vi "Teleop.vi"(10 "Match Info":T2={"Autonomous Elapsed Seconds"=0.0, "TeleOp Elapsed Seconds"=0.0, "Disabled Elapsed Seconds"=0.0, "Visited Autonomous"=FALSE, "Visited TeleOp"=FALSE, "Visited Disabled"=FALSE, "Autonomous Settings"={"Autonomous Style"=enum."Independent", "VI Refnum"=refnum}}, 11 "Call Context":T3) -> ()   [LabVIEW 2019]
doc: "This VI is called for each TeleOp packet received from the DS where the robot is not disabled. It is often used to read from the joysticks and update I/O or to update setpoints for timed control loops. It should complete and return within 20 milliseconds or it may miss DS packets."
uses:
  <vilib>/Rock Robotics/WPI/DriverStation/WPI_DriverStationDerivedRobotMode.ctl
  <vilib>/Rock Robotics/WPI/DriverStation/WPI_DriverStationMatch Info.ctl
  <vilib>/Rock Robotics/WPI/Solenoid/WPI_SolenoidValue.ctl
  <vilib>/Rock Robotics/WPI/Relay/WPI_RelayValue.ctl
  <vilib>/Rock Robotics/WPI/Utilities/WPI_GetSetVariantRefNum.vi
  <vilib>/Rock Robotics/Network Tables/NT Read Boolean.vi
  <vilib>/Rock Robotics/Network Tables/NT Write Boolean.vi
  <vilib>/Rock Robotics/WPI/RobotDrive/WPI_RobotDriveMecanumDrive_Cartesian.vi
  <vilib>/Rock Robotics/WPI/Solenoid/WPI_SolenoidSetEnum.vi
panel:
  out "Right JS\nButton 4\nConveyor\nReverse":bool
  out "Left JS\nButton 3\nCW Turner R override":bool
  out "Left JS\nButton 5\nCW Turner F override":bool
  out "FMS = Green":bool
  out "FMS = Yellow":bool
  out "FMS=Red":bool
  out "FMS=Blue":bool
  out "CW Turner Distance (in)":dbl
  out "Number of Revolutions":dbl
  out "Current angle (deg)":dbl
  out "Encoder Direction":dbl
  out "Encoder Rate (deg/sec)":dbl
  out "Left JS\nButton 8\nReset Encoder":bool
  out "Right JS\nButton 6\nConveyor\nForward":bool
  out "Right JS\nButton 1\nShooter":bool
  out "Button 4\nHD Off":bool
  out "Left JS Button 7\nCW Turner":bool
  out "Left JS\nButton 1\nWinch":bool
  out "Pincher Solenoid Value":T1
  out "Pincher Button Pressed":dbl
  out "Hook Deployer Solenoid Value":T1=enum."Forward"
  out "Hook Deployer \nButton Pressed":dbl
  out "Z value":dbl
  out "Y value":dbl
  out "X value":dbl
  out "Button 11\nPincher Release":bool
  out "Button 10\nPincher Off":bool
  out "Button 7\nPincher Grab":bool
  out "Button 5\nHD Up":bool
  out "Button 3\nHD Down":bool
  # "Drive Control"
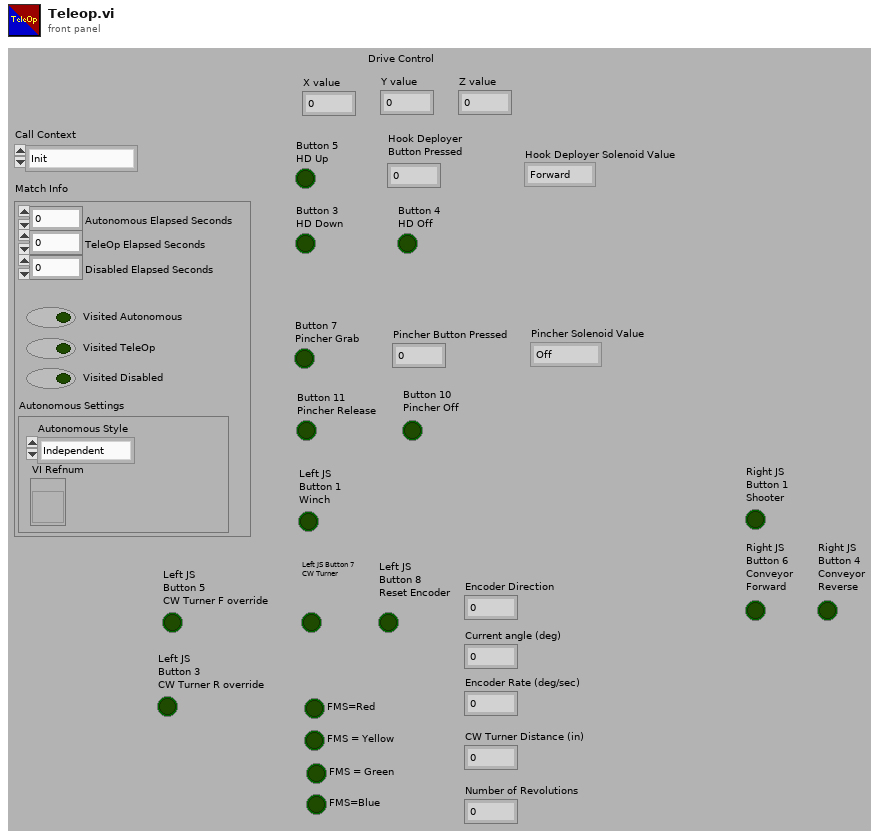
[diagram p1: front panel]
types:
  T1 = typedef "WPI_SolenoidValue.ctl" = enum16{"Off", "On", "Forward", "Reverse"}
  T2 = typedef "WPI_DriverStationMatch Info.ctl" = cluster{"Autonomous Elapsed Seconds":dbl, "TeleOp Elapsed Seconds":dbl, "Disabled Elapsed Seconds":dbl, "Visited Autonomous":bool, "Visited TeleOp":bool, "Visited Disabled":bool, "Autonomous Settings":cluster{"Autonomous Style":enum16{"Iterative", "Independent"}, "VI Refnum":refnum<vi>}}
  T3 = typedef "WPI_DriverStationDerivedRobotMode.ctl" = enum16{"Init", "Execute", "Stop"}
  T4 = typedef "WPI_EncoderDevRef.ctl" = cluster{"DevStatus":errorcluster, "EncoderIndex":T5, "CounterIndex":T6, "DistancePerCount":dbl, "Decoding Type":T7}
  T5 = typedef "FPGA_EncoderIdx.ctl" = enum8{"Enc 0", "Enc 1", "Enc 2", "Enc 3", "Enc 4", "Enc 5", "Enc 6", "Enc 7", "Invalid"}
  T6 = typedef "FPGA_CounterCtrSystemIndex.ctl" = enum8{"Ctr 0", "Ctr 1", "Ctr 2", "Ctr 3", "Ctr 4", "Ctr 5", "Ctr 6", "Ctr 7", "Invalid"}
  T7 = typedef "WPI_EncoderType.ctl" = enum16{"1x", "2x", "4x"}
  T8 = typedef "WPI_JoystickDevRef.ctl" = cluster{"Device":T9}
  T9 = typedef "WPI_JoystickDeviceEnum.ctl" = enum16{"USB 0", "USB 1", "USB 2", "USB 3", "USB 4", "USB 5"}
  T10 = typedef "WPI_RelayDevRef.ctl" = cluster{"DevStatus":errorcluster, "Relay Channel":T11, "Relay Direction":T12}
  T11 = typedef "FPGA_DIORelayChannel.ctl" = enum8{"Relay 0", "Relay 1", "Relay 2", "Relay 3", "Invalid"}
  T12 = typedef "WPI_RelayDirection.ctl" = enum16{"Both directions", "Forward only", "Reverse only"}
  T13 = typedef "WPI_RelayValue.ctl" = enum16{"Off", "On", "Forward", "Reverse"}
  T14 = typedef "WPI_MotorControlDeviceRef.ctl" = cluster{"DeviceStatus":errorcluster, "Type":T15, "PWM":cluster{"PWM Channel":T16, "DeadBand":T17}, "CAN":cluster{"Device Number":u8, "SetOutput VI Ref":variant, "GetOutput VI Ref":variant, "Enable VI Ref":variant, "Disable VI Ref":variant, "Data":variant}, "Invert":bool, "DIO PWM":cluster{"PWM \"Enable\" Channel":T16, "DIOChannel":T18, "PWM Rate":dbl}}
  T15 = typedef "WPI_MotorControlType.ctl" = enum16{"PWM", "CAN", "DIO PWM"}
  T16 = typedef "FPGA_DIOPWMChannel.ctl" = enum8{"PWM 0", "PWM 1", "PWM 2", "PWM 3", "PWM 4", "PWM 5", "PWM 6", "PWM 7", "PWM 8", "PWM 9", "PWM MXP 0", "PWM MXP 1", "PWM MXP 2", "PWM MXP 3", "PWM MXP 4", "PWM MXP 5", "PWM MXP 6", "PWM MXP 7", "PWM MXP 8", "PWM MXP 9", "Invalid"}
  T17 = typedef "WPI_PWMDeadband.ctl" = cluster{"Name":string, "maxPositivePwm":i32, "minPositivePwm":i32, "centerPwm":i32, "maxNegativePwm":i32, "minNegativePwm":i32, "angularRange":u16}
  T18 = typedef "FPGA_DIOChannel.ctl" = enum8{"DIO 0", "DIO 1", "DIO 2", "DIO 3", "DIO 4", "DIO 5", "DIO 6", "DIO 7", "DIO 8", "DIO 9", "DIO MXP 0", "DIO MXP 1", "DIO MXP 2", "DIO MXP 3", "DIO MXP 4", "DIO MXP 5", "DIO MXP 6", "DIO MXP 7", "DIO MXP 8", "DIO MXP 9", "DIO MXP 10", "DIO MXP 11", "DIO MXP 12", "DIO MXP 13", "DIO MXP 14", "DIO MXP 15", "SPI Port CS1", "SPI Port CS2", "SPI Port CS3", "SPI Port MISO", "SPI Port MOSI", "Invalid"}
  T19 = typedef "WPI_RobotDriveDevRef.ctl" = cluster{"DevStatus":errorcluster, "Motors[]":T14[], "Square Inputs":bool, "Max Output":dbl}
  T20 = typedef "WPI_SolenoidDevRef.ctl" = cluster{"DevStatus":errorcluster, "Pneumatics Control Module":u8, "Forward Solenoid Channel":T21, "Reverse Solenoid Channel":T21}
  T21 = typedef "WPI_SolenoidChannel.ctl" = enum8{"Solenoid 0", "Solenoid 1", "Solenoid 2", "Solenoid 3", "Solenoid 4", "Solenoid 5", "Solenoid 6", "Solenoid 7", "Invalid"}
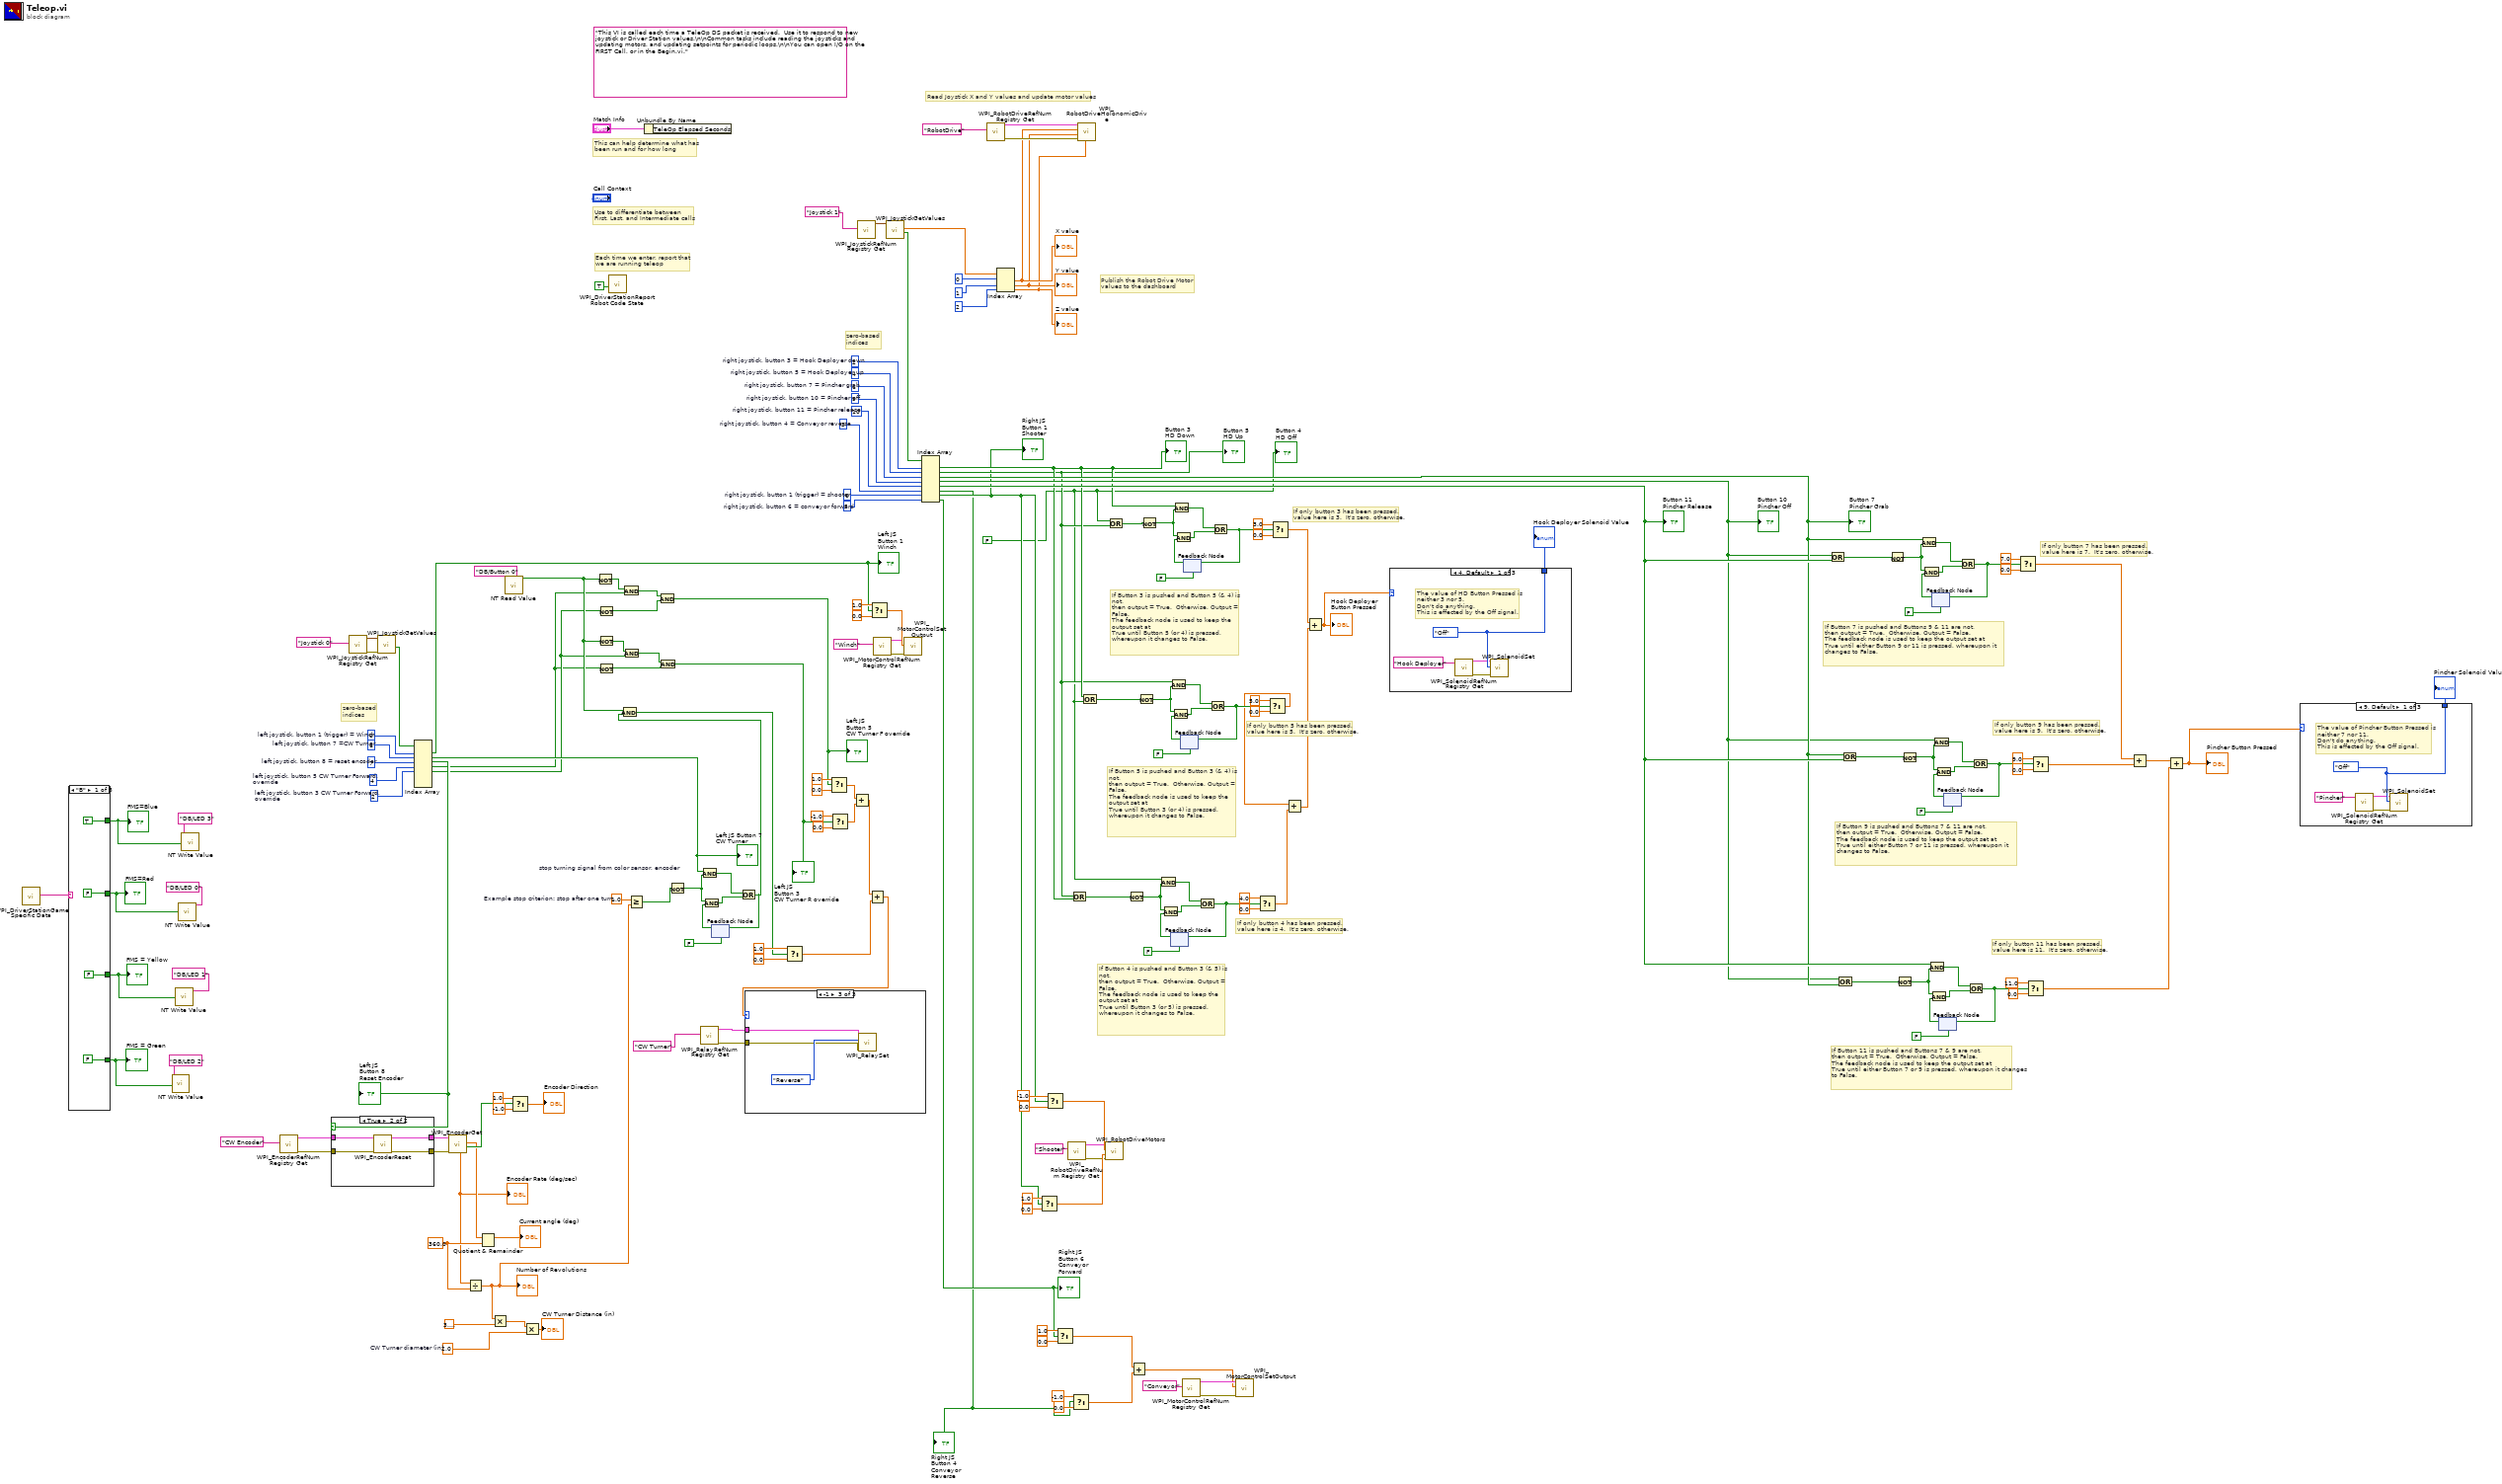
[diagram p0: block diagram]
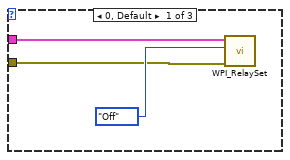
[diagram p2: hidden frame]
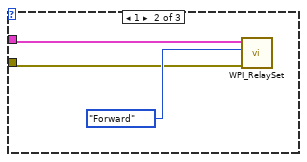
[diagram p3: hidden frame]
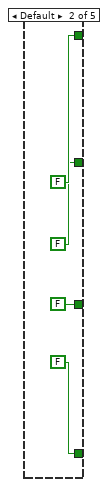
[diagram p4: hidden frame]
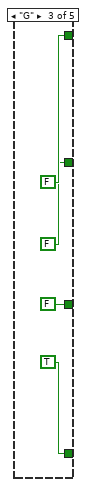
[diagram p5: hidden frame]
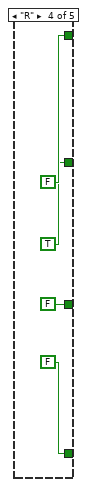
[diagram p6: hidden frame]
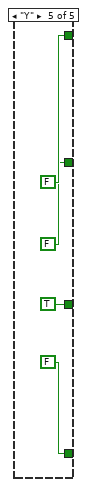
[diagram p7: hidden frame]
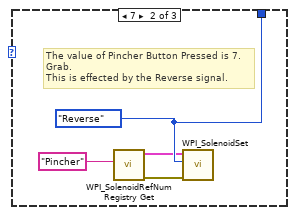
[diagram p9: hidden frame]
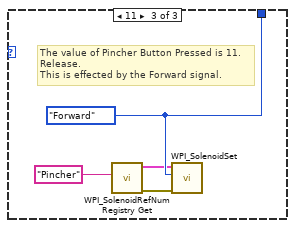
[diagram p10: hidden frame]
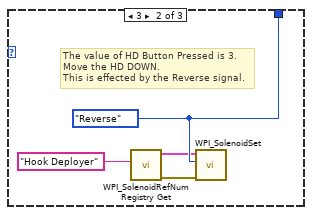
[diagram p11: hidden frame]
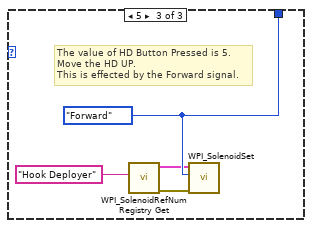
[diagram p12: hidden frame]
diagram:
  w7 = FALSE
  w34 = 2  # left joystick, button 3 CW Turner Forward, override
  w35 = 4  # left joystick, button 5 CW Turner Forward, override
  w62 = 1.0  # Example stop criterion: stop after one turn.
  w64 = 2.0  # CW Turner diameter (in)
  w69 = 360.0 ("y")
  w78 = 7  # left joystick, button 8 = reset encoder
  w88 = 5  # right joystick, button 6 = conveyor forward
  w89 = 0  # right joystick, button 1 (trigger) = shooter
  w106 = 3  # right joystick, button 4 = Conveyor reverse
  w119 = 6  # left joystick, button 7 =CW Turner
  w120 = 0  # left joystick, button 1 (trigger) = Winch
  w188 = 10  # right joystick, button 11 = Pincher release
  w189 = 9  # right joystick, button 10 = Pincher off
  w187 = 6  # right joystick, button 7 = Pincher grab
  w190 = 4  # right joystick, button 5 = Hook Deployer up
  w191 = 2  # right joystick, button 3 = Hook Deployer down
  (unwired) "This VI is called each time a TeleOp DS packet is received.  Use it to respond to new joystick or Driver Station values.\n\nCommon tasks include reading the joysticks and updating motors, and updating setpoints for periodic loops.\n\nYou can open I/O on the FIRST Call, or in the Begin.vi."
  # "If only button 4 has been pressed,\nvalue here is 4.  It's zero, otherwise."
  # "If Button 4 is pushed and Button 3 (& 5) is not,\nthen output = True.  Otherwise, Output = False.\nThe feedback node is used to keep the output set at \nTrue until Button 3 (or 5) is pressed, whereupon it changes to False."
  # "zero-based\nindices"
  # "zero-based\nindices"
  # "If only button 11 has been pressed,\nvalue here is 11.  It's zero, otherwise."
  # "If Button 11 is pushed and Buttons 7 & 9 are not,\nthen output = True.  Otherwise, Output = False.\nThe feedback node is used to keep the output set at \nTrue until either Button 7 or 9 is pressed, whereupon it changes to False."
  # "If only button 9 has been pressed,\nvalue here is 9.  It's zero, otherwise."
  # "If Button 9 is pushed and Buttons 7 & 11 are not,\nthen output = True.  Otherwise, Output = False.\nThe feedback node is used to keep the output set at \nTrue until either Button 7 or 11 is pressed, whereupon it changes to False."
  # "If only button 7 has been pressed,\nvalue here is 7.  It's zero, otherwise."
  # "If Button 7 is pushed and Buttons 9 & 11 are not,\nthen output = True.  Otherwise, Output = False.\nThe feedback node is used to keep the output set at \nTrue until either Button 9 or 11 is pressed, whereupon it changes to False."
  # "If only button 5 has been pressed,\nvalue here is 5.  It's zero, otherwise."
  # "If only button 3 has been pressed,\nvalue here is 3.  It's zero, otherwise."
  # "If Button 5 is pushed and Button 3 (& 4) is not,\nthen output = True.  Otherwise, Output = False.\nThe feedback node is used to keep the output set at \nTrue until Button 3 (or 4) is pressed, whereupon it changes to False."
  # "If Button 3 is pushed and Button 5 (& 4) is not,\nthen output = True.  Otherwise, Output = False.\nThe feedback node is used to keep the output set at \nTrue until Button 5 (or 4) is pressed, whereupon it changes to False."
  # "Publish the Robot Drive Motor\nvalues to the dashboard"
  # "Each time we enter, report that\nwe are running teleop"
  # "Use to differentiate between\nFirst, Last, and Intermediate calls"
  # "This can help determine what has\nbeen run and for how long"
  # "Read Joystick X and Y values and update motor values"
  n1 = call <vilib>:"WPI_DriverStationGame Specific Data.vi"() -> ("Game Specific Data"=w44:string)  [unwired: 11 in]
  n2 = case shown="\"B\"" w44 {
    tunnel: [TRUE ("FMS=Blue") FALSE ("FMS=Blue") FALSE ("FMS=Blue") FALSE ("FMS=Blue") FALSE ("FMS=Blue")] -> w42
    tunnel: [FALSE ("FMS=Blue") FALSE ("FMS=Blue") FALSE ("FMS=Blue") TRUE ("FMS=Blue") FALSE ("FMS=Blue")] -> w39
    tunnel: [FALSE ("FMS=Blue") FALSE ("FMS=Blue") FALSE ("FMS=Blue") FALSE ("FMS=Blue") TRUE ("FMS=Blue")] -> w36
    tunnel: [FALSE ("FMS=Blue") FALSE ("FMS=Blue") TRUE ("FMS=Blue") FALSE ("FMS=Blue") FALSE ("FMS=Blue")] -> w40
    frame "B" {
    }
    frame Default {
    }
    frame "G" {
    }
    frame "R" {
    }
    frame "Y" {
    }
  }
  "FMS=Blue" <- w42
  "FMS=Red" <- w39
  "FMS = Yellow" <- w36
  "FMS = Green" <- w40
  n3 = call-poly <vilib>:"NT Write Value.vi"("Boolean"=w40, "Name"="DB/LED 2") -> ()  [unwired: 9 in, 1 out]
  n4 = call-poly <vilib>:"NT Write Value.vi"("Boolean"=w36, "Name"="DB/LED 1") -> ()  [unwired: 9 in, 1 out]
  n5 = call-poly <vilib>:"NT Write Value.vi"("Boolean"=w39, "Name"="DB/LED 0") -> ()  [unwired: 9 in, 1 out]
  n6 = call-poly <vilib>:"NT Write Value.vi"("Boolean"=w42, "Name"="DB/LED 3") -> ()  [unwired: 9 in, 1 out]
  n7 = call <vilib>:"WPI_EncoderRefNum Registry Get.vi"("refnum name"="CW Encoder") -> ("error out"=w59:errorcluster, "EncoderDevRef"=w60:T4)  [unwired: 9 in]
  n8 = call <vilib>:"WPI_JoystickRefNum Registry Get.vi"("refnum name"="Joystick 0") -> ("error out"=w107:errorcluster, "JoystickDevRef"=w182:T8)  [unwired: 1 in, 8 out]
  n9 = call <vilib>:"WPI_JoystickGetValues.vi"("error in (no error)"=w107, "JoystickDevRef"=w182) -> ("Buttons"=w118:bool[])  [unwired: 5 in, 4 out]
  n10 = Index Array(array=w118, index #1=w120, index #2=w119, index #3=w78, index #4=w35, index #5=w34) -> (element #1=w48:bool, element #2=w47:bool, element #3=w46:bool, element #4=w14:bool, element #5=w15:bool)  [unwired: 3 in, 3 out]
  "Left JS\nButton 1\nWinch" <- w48
  "Left JS Button 7\nCW Turner" <- w47
  "Left JS\nButton 8\nReset Encoder" <- w46
  n11 = case shown="True" w46 {
    tunnel: w60 -> [w219 w223]
    tunnel: [w219 w222] -> w77
    tunnel: w59 -> [w218 w221]
    tunnel: [w218 w220] -> w76
    frame False {
    }
    frame True {
      n12 = call <vilib>:"WPI_EncoderReset.vi"("error in (no error)"=w221, "EncoderDevRef"=w223) -> ("error out"=w220:errorcluster, "EncoderDevRef"=w222:T4)  [unwired: 8 in]
    }
  }
  n13 = call <vilib>:"WPI_EncoderGet.vi"("error in (no error)"=w76, "EncoderDevRef"=w77) -> ("Direction"=w74:bool, "Distance"=w71:dbl, "Rate"=w68:dbl)  [unwired: 4 in, 3 out]
  "Encoder Rate (deg/sec)" <- w68
  n14 = Divide(x=w68, y=w69) -> (x/y=w61:dbl)
  "Number of Revolutions" <- w61
  n15 = Quotient & Remainder(x=w71, y=w69) -> (x-y*floor(x/y)=→"Current angle (deg)":dbl)  [unwired: 1 out]
  n16 = Multiply(x=w61, y=3.141592653589793) -> (x*y=w66:dbl)
  n17 = call-poly <vilib>:"NT Read Value.vi"("Name"="DB/Button 0") -> ("Boolean"=w18:bool)  [unwired: 9 in, 1 out]
  n18 = Select(t=1.0, s=w74, f=-1.0) -> (s? t:f=→"Encoder Direction":dbl)
  n19 = Multiply(x=w66, y=w64) -> (x*y=→"CW Turner Distance (in)":dbl)
  n20 = Not(x=w18) -> (.not. x?=w19:bool)
  n21 = Not(x=w15) -> (.not. x?=w13:bool)
  n22 = Not(x=w18) -> (.not. x?=w20:bool)
  n23 = Not(x=w14) -> (.not. x?=w11:bool)
  n24 = call <vilib>:"WPI_DriverStationReport Robot Code State.vi"("TeleOp"=TRUE ("Autonomous")) -> ()  [unwired: 10 in, 1 out]
  n25 = And(x=w19, y=w14) -> (x .and. y?=w12:bool)
  n26 = And(x=w20, y=w15) -> (x .and. y?=w10:bool)
  n27 = Greater Or Equal?(x=w62, y=w61) -> (x >= y?=w63:bool)
  n28 = Unbundle By Name("Match Info") -> ()  [unwired: 1 out]
  n29 = And(x=w12, y=w13) -> (x .and. y?=w9:bool)
  "Left JS\nButton 5\nCW Turner F override" <- w9
  n30 = And(x=w10, y=w11) -> (x .and. y?=w8:bool)
  "Left JS\nButton 3\nCW Turner R override" <- w8
  n31 = Not "stop turning signal from color sensor, encoder"(x=w63) -> (.not. x?=w112:bool)
  n32 = And(x=w47, y=w112) -> (x .and. y?=w111:bool)
  n33 = call <vilib>:"WPI_RelayRefNum Registry Get.vi"("refnum name"="CW Turner") -> ("error out"=w22:errorcluster, "RelayDevRef"=w21:T10)  [unwired: 9 in]
  n34 = feedback #1(FALSE) -> (w109:bool)
  n35 = And(x=w112, y=w109) -> (x .and. y?=w110:bool)
  n36 = Or(x=w111, y=w110) -> (x .or. y?=w17:bool)
  n37 = And(x=w18, y=w17) -> (x .and. y?=w16:bool)
  n38 = feedback-in #1(w17) -> ()
  n39 = Select(t=1.0, s=w16, f=0.0) -> (s? t:f=w27:dbl)
  n40 = Select(t=1.0, s=w9, f=0.0) -> (s? t:f=w29:dbl)
  n41 = Select(t=-1.0, s=w8, f=0.0) -> (s? t:f=w28:dbl)
  n42 = Add(x=w29, y=w28) -> (x+y=w26:dbl)
  n43 = call <vilib>:"WPI_JoystickRefNum Registry Get.vi"("refnum name"="Joystick 1") -> ("JoystickDevRef"=w195:T8)  [unwired: 1 in, 9 out]
  n44 = Add(x=w26, y=w27) -> (x+y=w24:dbl)
  n45 = case shown="-1" w24 {
    tunnel: w22 -> [w225 w227 w230]
    tunnel: w21 -> [w224 w228 w231]
    frame 0, Default {
      n46 = call <vilib>:"WPI_RelaySet.vi"("error in (no error)"=w225, "RelayValue"=WPI_RelayValue."Off", "RelayDevRef"=w224) -> ()  [unwired: 7 in, 2 out]
    }
    frame 1 {
      n47 = call <vilib>:"WPI_RelaySet.vi"("error in (no error)"=w227, "RelayValue"=WPI_RelayValue."Forward", "RelayDevRef"=w228) -> ()  [unwired: 7 in, 2 out]
    }
    frame -1 {
      n48 = call <vilib>:"WPI_RelaySet.vi"("error in (no error)"=w230, "RelayValue"=WPI_RelayValue."Reverse", "RelayDevRef"=w231) -> ()  [unwired: 7 in, 2 out]
    }
  }
  n49 = Select(t=1.0, s=w48, f=0.0) -> (s? t:f=w117:dbl)
  n50 = call <vilib>:"WPI_MotorControlRefNum Registry Get.vi"("refnum name"="Winch") -> ("error out"=w55:errorcluster, "MotorControlDevRef"=w56:T14)  [unwired: 9 in]
  n51 = call <vilib>:"WPI_JoystickGetValues.vi"("JoystickDevRef"=w195) -> ("Buttons"=w192:bool[], "Axes"=w193:dbl[])  [unwired: 6 in, 3 out]
  n52 = call <vilib>:"WPI_MotorControlSetOutput.vi"("error in (no error)"=w55, "Output"=w117, "MotorControlDevRef"=w56) -> ()  [unwired: 6 in, 3 out]
  n53 = Index Array(array=w192, index #1=w191, index #2=w190, index #3=w187, index #4=w189, index #5=w188, index #6=w106, index #7=w89, index #8=w88) -> (element #1=w94:bool, element #2=w93:bool, element #3=w122:bool, element #4=w121:bool, element #5=w123:bool, element #6=w4:bool, element #7=w45:bool, element #8=w79:bool)
  "Button 3\nHD Down" <- w94
  "Button 5\nHD Up" <- w93
  "Button 7\nPincher Grab" <- w122
  "Button 10\nPincher Off" <- w121
  "Button 11\nPincher Release" <- w123
  "Right JS\nButton 1\nShooter" <- w45
  "Right JS\nButton 6\nConveyor\nForward" <- w79
  "Right JS\nButton 4\nConveyor\nReverse" <- w4
  n54 = call <vilib>:"WPI_RobotDriveRefNum Registry Get.vi"("refnum name"="RobotDrive") -> ("error out"=w179:errorcluster, "RobotDriveDevRef"=w180:T19)  [unwired: 9 in]
  n55 = Index Array(array=w193, index #1=0 ("index"), index #2=1 ("index"), index #3=2 ("index")) -> (element #1=w178:dbl, element #2=w177:dbl, element #3=w176:dbl)
  "X value" <- w178
  "Y value" <- w177
  "Z value" <- w176
  n56 = Select(t=1.0, s=w45, f=0.0) -> (s? t:f=w82:dbl)
  n57 = Select(t=-1.0, s=w45, f=0.0) -> (s? t:f=w85:dbl)
  n58 = Select(t=1.0, s=w79, f=0.0) -> (s? t:f=w2:dbl)
  n59 = call <vilib>:"WPI_RobotDriveRefNum Registry Get.vi"("refnum name"="Shooter") -> ("error out"=w52:errorcluster, "RobotDriveDevRef"=w53:T19)  [unwired: 9 in]
  n60 = Or(x=w93, y=w94) -> (x .or. y?=w95:bool)
  n61 = Select(t=-1.0, s=w4, f=0.0) -> (s? t:f=w3:dbl)
  n62 = call-poly <vilib>:"WPI_RobotDriveHolonomicDrive.vi"("Rotation"=w176, "error in (no error)"=w179, "Y"=w177, "X"=w178, "RobotDriveDevRef"=w180) -> ()  [unwired: 4 in, 3 out]
  n63 = Or(x=w94, y=w7) -> (x .or. y?=w104:bool)
  n64 = call <vilib>:"WPI_RobotDriveMotors.vi"("error in (no error)"=w52, "RightSpeed"=w82, "LeftSpeed"=w85, "RobotDriveDevRef"=w53) -> ()  [unwired: 5 in, 3 out]
  n65 = Or(x=w7, y=w93) -> (x .or. y?=w105:bool)
  n66 = Not(x=w95) -> (.not. x?=w103:bool)
  n67 = Add(x=w2, y=w3) -> (x+y=w1:dbl)
  n68 = Not(x=w104) -> (.not. x?=w169:bool)
  n69 = Not(x=w105) -> (.not. x?=w175:bool)
  n70 = And(x=w7, y=w103) -> (x .and. y?=w102:bool)
  n71 = And(x=w93, y=w169) -> (x .and. y?=w168:bool)
  n72 = feedback #2(FALSE) -> (w100:bool)
  n73 = And(x=w103, y=w100) -> (x .and. y?=w101:bool)
  n74 = And(x=w94, y=w175) -> (x .and. y?=w174:bool)
  n75 = feedback #3(FALSE) -> (w166:bool)
  n76 = And(x=w169, y=w166) -> (x .and. y?=w167:bool)
  n77 = call <vilib>:"WPI_MotorControlRefNum Registry Get.vi"("refnum name"="Conveyor") -> ("error out"=w50:errorcluster, "MotorControlDevRef"=w51:T14)  [unwired: 9 in]
  n78 = feedback #4(FALSE) -> (w172:bool)
  n79 = And(x=w175, y=w172) -> (x .and. y?=w173:bool)
  n80 = Or(x=w102, y=w101) -> (x .or. y?=w98:bool)
  n81 = feedback-in #2(w98) -> ()
  n82 = Or(x=w168, y=w167) -> (x .or. y?=w164:bool)
  n83 = feedback-in #3(w164) -> ()
  n84 = Or(x=w174, y=w173) -> (x .or. y?=w170:bool)
  n85 = feedback-in #4(w170) -> ()
  n86 = call <vilib>:"WPI_MotorControlSetOutput.vi"("error in (no error)"=w50, "Output"=w1, "MotorControlDevRef"=w51) -> ()  [unwired: 6 in, 3 out]
  n87 = Select(t=4.0, s=w98, f=0.0) -> (s? t:f=w92:dbl)
  n88 = Select(t=5.0, s=w164, f=0.0) -> (s? t:f=w91:dbl)
  n89 = Select(t=3.0, s=w170, f=0.0) -> (s? t:f=w159:dbl)
  n90 = Add(x=w91, y=w92) -> (x+y=w90:dbl)
  n91 = Add(x=w159, y=w90) -> (x+y=w158:dbl)
  "Hook Deployer \nButton Pressed" <- w158
  n92 = case shown="4, Default" w158 {
    tunnel: [w236 w240 w244] -> w157
    frame 4, Default {
      w236 = WPI_SolenoidValue."Off" ("Value")
      # "The value of HD Button Pressed is \nneither 3 nor 5.\nDon't do anything.\nThis is effected by the Off signal."
      n93 = call <vilib>:"WPI_SolenoidRefNum Registry Get.vi"("refnum name"="Hook Deployer") -> ("error out"=w235:errorcluster, "SolenoidDevRef"=w234:T20)  [unwired: 9 in]
      n94 = call-poly <vilib>:"WPI_SolenoidSet.vi"("error in (no error)"=w235, "Value"=w236, "SolenoidDevRef"=w234) -> ()  [unwired: 7 in, 2 out]
    }
    frame 3 {
      w240 = WPI_SolenoidValue."Reverse" ("Value")
      # "The value of HD Button Pressed is 3.\nMove the HD DOWN.\nThis is effected by the Reverse signal."
      n95 = call <vilib>:"WPI_SolenoidRefNum Registry Get.vi"("refnum name"="Hook Deployer") -> ("error out"=w237:errorcluster, "SolenoidDevRef"=w238:T20)  [unwired: 9 in]
      n96 = call-poly <vilib>:"WPI_SolenoidSet.vi"("error in (no error)"=w237, "Value"=w240, "SolenoidDevRef"=w238) -> ()  [unwired: 7 in, 2 out]
    }
    frame 5 {
      w244 = WPI_SolenoidValue."Forward" ("Value")
      # "The value of HD Button Pressed is 5.\nMove the HD UP.\nThis is effected by the Forward signal."
      n97 = call <vilib>:"WPI_SolenoidRefNum Registry Get.vi"("refnum name"="Hook Deployer") -> ("error out"=w241:errorcluster, "SolenoidDevRef"=w242:T20)  [unwired: 9 in]
      n98 = call-poly <vilib>:"WPI_SolenoidSet.vi"("error in (no error)"=w241, "Value"=w244, "SolenoidDevRef"=w242) -> ()  [unwired: 7 in, 2 out]
    }
  }
  "Hook Deployer Solenoid Value" <- w157
  n99 = Or(x=w121, y=w123) -> (x .or. y?=w147:bool)
  n100 = Or(x=w121, y=w122) -> (x .or. y?=w129:bool)
  n101 = Or(x=w122, y=w123) -> (x .or. y?=w138:bool)
  n102 = Not(x=w147) -> (.not. x?=w156:bool)
  n103 = Not(x=w129) -> (.not. x?=w137:bool)
  n104 = Not(x=w138) -> (.not. x?=w146:bool)
  n105 = And(x=w122, y=w156) -> (x .and. y?=w155:bool)
  n106 = And(x=w123, y=w137) -> (x .and. y?=w136:bool)
  n107 = feedback #5(FALSE) -> (w153:bool)
  n108 = And(x=w156, y=w153) -> (x .and. y?=w154:bool)
  n109 = And(x=w121, y=w146) -> (x .and. y?=w145:bool)
  n110 = feedback #6(FALSE) -> (w134:bool)
  n111 = And(x=w137, y=w134) -> (x .and. y?=w135:bool)
  n112 = feedback #7(FALSE) -> (w143:bool)
  n113 = And(x=w146, y=w143) -> (x .and. y?=w144:bool)
  n114 = Or(x=w155, y=w154) -> (x .or. y?=w151:bool)
  n115 = feedback-in #5(w151) -> ()
  n116 = Or(x=w136, y=w135) -> (x .or. y?=w132:bool)
  n117 = feedback-in #6(w132) -> ()
  n118 = Or(x=w145, y=w144) -> (x .or. y?=w141:bool)
  n119 = feedback-in #7(w141) -> ()
  n120 = Select(t=7.0, s=w151, f=0.0) -> (s? t:f=w148:dbl)
  n121 = Select(t=11.0, s=w132, f=0.0) -> (s? t:f=w126:dbl)
  n122 = Select(t=9.0, s=w141, f=0.0) -> (s? t:f=w128:dbl)
  n123 = Add(x=w148, y=w128) -> (x+y=w127:dbl)
  n124 = Add(x=w127, y=w126) -> (x+y=w125:dbl)
  "Pincher Button Pressed" <- w125
  n125 = case shown="9, Default" w125 {
    tunnel: [w248 w252 w256] -> w124
    frame 9, Default {
      w248 = WPI_SolenoidValue."Off" ("Value")
      # "The value of Pincher Button Pressed is \nneither 7 nor 11.\nDon't do anything.\nThis is effected by the Off signal."
      n126 = call <vilib>:"WPI_SolenoidRefNum Registry Get.vi"("refnum name"="Pincher") -> ("error out"=w247:errorcluster, "SolenoidDevRef"=w246:T20)  [unwired: 9 in]
      n127 = call-poly <vilib>:"WPI_SolenoidSet.vi"("error in (no error)"=w247, "Value"=w248, "SolenoidDevRef"=w246) -> ()  [unwired: 7 in, 2 out]
    }
    frame 7 {
      w252 = WPI_SolenoidValue."Reverse" ("Value")
      # "The value of Pincher Button Pressed is 7.\nGrab.\nThis is effected by the Reverse signal."
      n128 = call <vilib>:"WPI_SolenoidRefNum Registry Get.vi"("refnum name"="Pincher") -> ("error out"=w249:errorcluster, "SolenoidDevRef"=w250:T20)  [unwired: 9 in]
      n129 = call-poly <vilib>:"WPI_SolenoidSet.vi"("error in (no error)"=w249, "Value"=w252, "SolenoidDevRef"=w250) -> ()  [unwired: 7 in, 2 out]
    }
    frame 11 {
      w256 = WPI_SolenoidValue."Forward" ("Value")
      # "The value of Pincher Button Pressed is 11.\nRelease.\nThis is effected by the Forward signal."
      n130 = call <vilib>:"WPI_SolenoidRefNum Registry Get.vi"("refnum name"="Pincher") -> ("error out"=w253:errorcluster, "SolenoidDevRef"=w254:T20)  [unwired: 9 in]
      n131 = call-poly <vilib>:"WPI_SolenoidSet.vi"("error in (no error)"=w253, "Value"=w256, "SolenoidDevRef"=w254) -> ()  [unwired: 7 in, 2 out]
    }
  }
  "Pincher Solenoid Value" <- w124
  "Button 4\nHD Off" <- w7
